vi "tsapp_transmit_lin_gotosleep_async.vi"(5 "AWakeupIntervalTime":i32, 7 "AWakeupTimes":i32, 8 "错误输入（无错误）":errorcluster, 9 "AWakeupLength":i32, 10 "ALdxChn":i32, 11 "路径输入":path) -> (0 "错误输出":errorcluster, 2 "return":i32, 3 "路径输出":path)   [LabVIEW 2014]
doc: "Function Introduction :\nAsynchronous sending of lin wake-up message\nCall location :\ninput parameter :\nAIdxChn: Channel Index\nAWakeupLength: wake-up message length\nAWakeupIntervalTime: Wake up interval\nAWakeupTimes: Wake up time\nReturn value :\n0: Execution successful\nOther values: Failed"
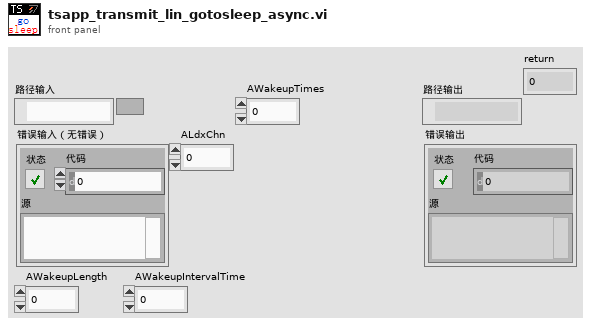
[diagram p1: front panel]
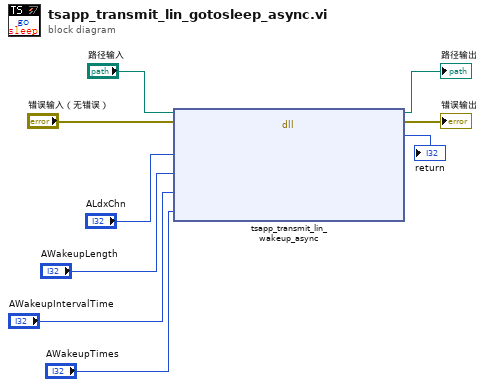
[diagram p0: block diagram]
diagram:
  n1 = dll-call lib="D:/Program Files (x86)/TOSUN/TSMaster/Data/SDK/lib/x86/TSMaster.dll" fn="tsapp_transmit_lin_wakeup_async"(path in="路径输入", error in="错误输入（无错误）", "ALdxChn"="ALdxChn", "AWakeupLength"="AWakeupLength", "AWakeupIntervalTime"="AWakeupIntervalTime", "AWakeupTimes"="AWakeupTimes") -> (path out=→"路径输出":path, error out=→"错误输出":errorcluster, "返回类型"=→"return":i32)  [unwired: 5 in]
